vi "Get SMO Public API.vi"(8 "error in (no error)":errorcluster, 11 "Inst.TC in":refnum<class "Inst.TC.lvclass">) -> (0 "error out":errorcluster, 2 "Commands":string[](array[string]), 3 "Inst.TC out":refnum<class "Inst.TC.lvclass">)   [LabVIEW 2019, in "Inst.TC.lvclass"]
uses:
  Inst.TC.lvclass
  Typedefs/Inst.TC.Commands--Enum.ctl
  98296d38-2bf1-4698-a8d3-81badd63a6cc.vi
  <vilib>/Utility/Data Type/Get Type Information.vi
  <vilib>/Utility/Data Type/Get Numeric Information.vi
  <userlib>/_OpenG.lib/lvdata/lvdata.llb/Unwrap VVariant__ogtk.vi
  <userlib>/LevyLab/Instrument Framework/Instrument Types/Cryostat/Instrument.Cryostat.lvclass
  <userlib>/LevyLab/Instrument Framework/Instrument/Instrument.lvclass
  C:/Program Files (x86)/National Instruments/LabVIEW 2019/user.lib/LevyLab/Instrument Framework/Instrument Types/Cryostat/Instrument.Cryostat.lvclass
  C:/Program Files (x86)/National Instruments/LabVIEW 2019/user.lib/LevyLab/Instrument Framework/Instrument/Instrument.lvclass
  C:/Program Files (x86)/National Instruments/LabVIEW 2019/vi.lib/JKI/JKI SMO/SMO/SMO.lvclass
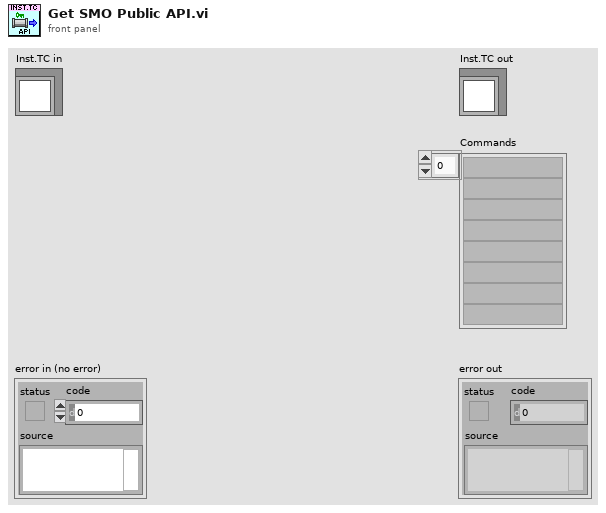
[diagram p1: front panel]
types:
  T1 = typedef "Inst.TC.lvclass/Inst.TC.Commands--Enum.ctl" = enum16{"getTemperature", "getHeater", "setHeater"}
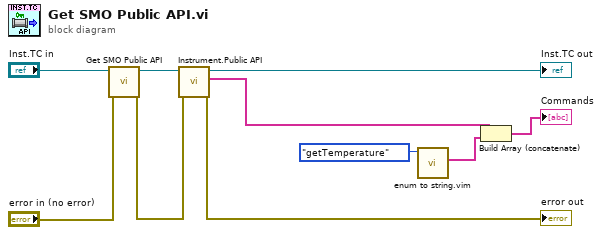
[diagram p0: block diagram]
diagram:
  n1 = call-parent "Get SMO Public API.vi"("error in (no error)"="error in (no error)", "Instrument.Cryostat in"="Inst.TC in") -> ("error out"=w2:errorcluster, "Instrument.Cryostat out"=w4:refnum<class "Inst.TC.lvclass">)  [unwired: 7 in, 1 out]
  n2 = call <userlib>:"Instrument.Public API.vi"("error in (no error)"=w2, "Instrument in"=w4) -> ("error out"=→"error out":errorcluster, "commands (this level)"=w5:string[], "Instrument out"=→"Inst.TC out":refnum<class "Inst.TC.lvclass">)  [unwired: 7 in]
  n3 = call "enum to string.vim"("enum in"=Inst.TC.Commands--Enum."getTemperature" ("Commands")) -> ("strings out"=w6:string[])  [unwired: 9 in, 1 out]
  n4 = Build Array (concatenate)(w5, w6) -> (→"Commands":string[])
